vi "CSM - Convert HexStr to Data.vi"(2 "HEX String":string, 3 "error in (no error)":errorcluster) -> (7 "Variant":variant, 9 "error out":errorcluster)   [LabVIEW 2017, in "Communicable State Machine.lvlib"]
doc: "Converts the hexadecimal string argument back to Variant data.\n\n\n> [!NOTE] <b>CSM Argument Type</b>\n>\n> In CSM, all arguments and return values are presented in string format, but they can carry any data type underneath. Therefore, the sender must encode first, and the receiver must decode afterwards. For example, CSM has a built-in HEXSTR encoding scheme, and custom codecs can also be extended as needed. To facilitate the identification of the encoding method, it is recommended to write the encoded argument in the format `<Argument Type> STRING FORMAT ARGUMENT`. Use the CSM - Argument Type VI to extract the type tag and select the corresponding decoding function accordingly.\n\n\n> [!NOTE] <b>CSM HEXSTR Format Argument</b>\n>\n> To pass arbitrary data types in CSM arguments, CSM has a built-in HEXSTR format argument encoding/decoding scheme. The argument type string is HEXSTR. The conversion process is as follows:\n>\n> 1. Convert LabVIEW data to a variant.\n> 2. Serialize the memory image of the variant into a hexadecimal string;\n> 3. Obtain the argument in the form `<HEXSTR> hexadecimal string`, which can be safely embedded in the state string without disrupting CSM message parsing.\n\n\n<b>Reference Example</b>: `[CSM-Example]\\0. Base Concepts\\4.1 Arguments - Complex Data As Arguments.vi`.\n\n-- <b>Controls</b> --\n- <b>HEX String</b>: CSM HEXSTR format argument.\n\n-- <b>Indicators</b> --\n- <b>Variant</b>: LabVIEW data. Supports any data type via Variant."
uses:
  Communicable State Machine.lvlib
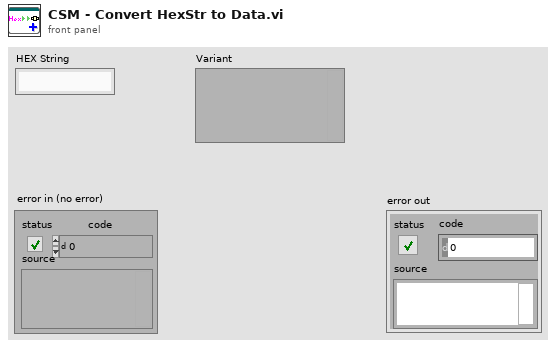
[diagram p1: front panel]
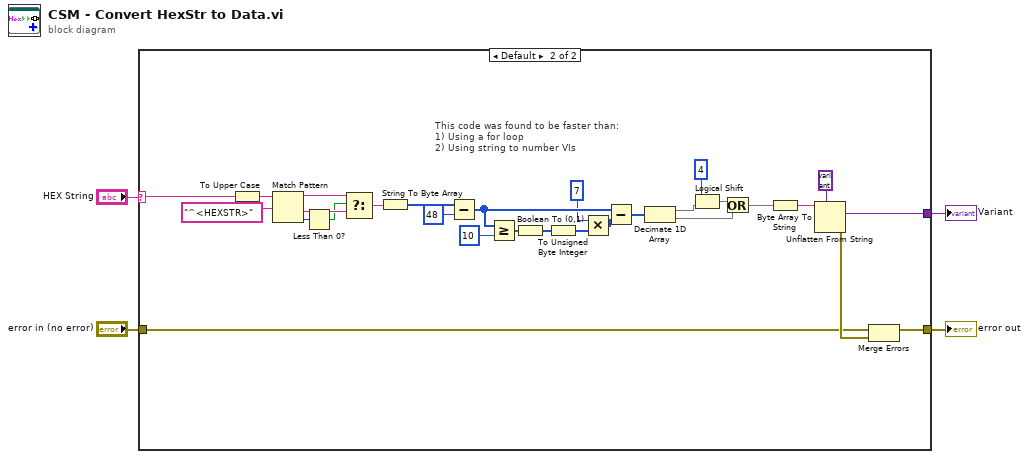
[diagram p0: block diagram]
diagram:
  n1 = case shown="Default" "HEX String" {
    selector: "HEX String" -> [_ w7]
    tunnel: [_ w33] -> w4
    tunnel: [w5 w15] -> w2
    tunnel: "error in (no error)" -> [w5 w14]
    frame "" {
    }
    frame Default {
      # "This code was found to be faster than:\n1) Using a for loop\n2) Using string to number VIs"
      n2 = To Upper Case(1:w7) -> (0:w13:string)
      n3 = Match Pattern(string=w13, regular expression="^<HEXSTR>") -> (before substring=w10:string, after substring=w9:string, offset past match=w11:i32)  [unwired: 1 in, 1 out]
      n4 = Less Than 0?(x=w11) -> (x < 0?=w8:bool)
      n5 = Select(t=w10, s=w8, f=w9) -> (s? t:f=w6:string)
      n6 = String To Byte Array(string=w6) -> (unsigned byte array=w18:u8[])
      n7 = Subtract(x=w18, y=u8 48) -> (x-y=w29:u8[])
      n8 = Greater Or Equal?(x=w29, y=u8 10) -> (x >= y?=w26:bool[])
      n9 = Boolean To (0,1)(Boolean=w26) -> (0, 1=w24:i16[])
      n10 = To Unsigned Byte Integer(number=w24) -> (unsigned 8bit integer=w27:u8[])
      n11 = Multiply(x=u8 7, y=w27) -> (x*y=w28:u8[])
      n12 = Subtract(x=w29, y=w28) -> (x-y=w20:u8[])
      n13 = Decimate 1D Array(w20) -> (w21:u8[], w19:u8[])
      n14 = Logical Shift(y=i8 4, x=w21) -> (x << y=w30:u8[])
      n15 = Or(x=w30, y=w19) -> (x .or. y?=w17:u8[])
      n16 = Byte Array To String(unsigned byte array=w17) -> (string=w32:string)
      n17 = Unflatten From String(type=variant, binary string=w32) -> (value=w33:variant, error out=w16:errorcluster)  [unwired: 3 in, 1 out]
      n18 = Merge Errors(w14, w16) -> (w15:errorcluster)
    }
  }
  "Variant" <- w4
  "error out" <- w2
